vi "4 - extract full movement patterns from XY frame and startend frames.vi"() -> ()   [LabVIEW 2013]
uses:
  <vilib>/Utility/file.llb/Read From Spreadsheet File (DBL).vi
panel:
  in  "XY and frame data 2":path
  in  "Startend":path
  in  "Player position segment data":path
  out "Sub patterns top":string[](array[string])
  out "Sub patterns bottom":string[](array[string])
  out "top":string[](array[string])
  out "bottom":string[](array[string])
  in  "player transition data":dbl[][](array[numeric])=array14018x2[28036 elements] format="%0.3f"
  in  "startend":dbl[][](array[numeric])=[[400.0, 872.0], [1216.0, 1280.0], [1504.0, 1664.0], [2584.0, 2648.0], [2944.0, 3128.0], [3440.0, 3512.0], [3752.0, 4232.0], [4696.0, 4816.0], [5392.0, 5624.0], [6008.0, 6296.0], [6736.0, 7016.0], [7344.0, 7864.0], [8368.0, 8464.0], [8864.0, 8992.0], [9320.0, 9704.0], [11288.0, 11432.0], [11768.0, 11872.0], [12256.0, 12536.0], [12888.0, 13024.0], [13520.0, 13632.0], [13856.0, 14000.0], [14208.0, 14304.0], [14600.0, 14792.0], [15280.0, 15416.0], [15648.0, 15760.0], [16672.0, 16800.0], [17008.0, 17224.0], [17536.0, 17664.0], [17936.0, 18144.0], [18392.0, 18568.0]] format="%0.3f"
  in  "XY and frame data":dbl[][](array[numeric])=array14019x5[70095 elements] format="%0.3f"
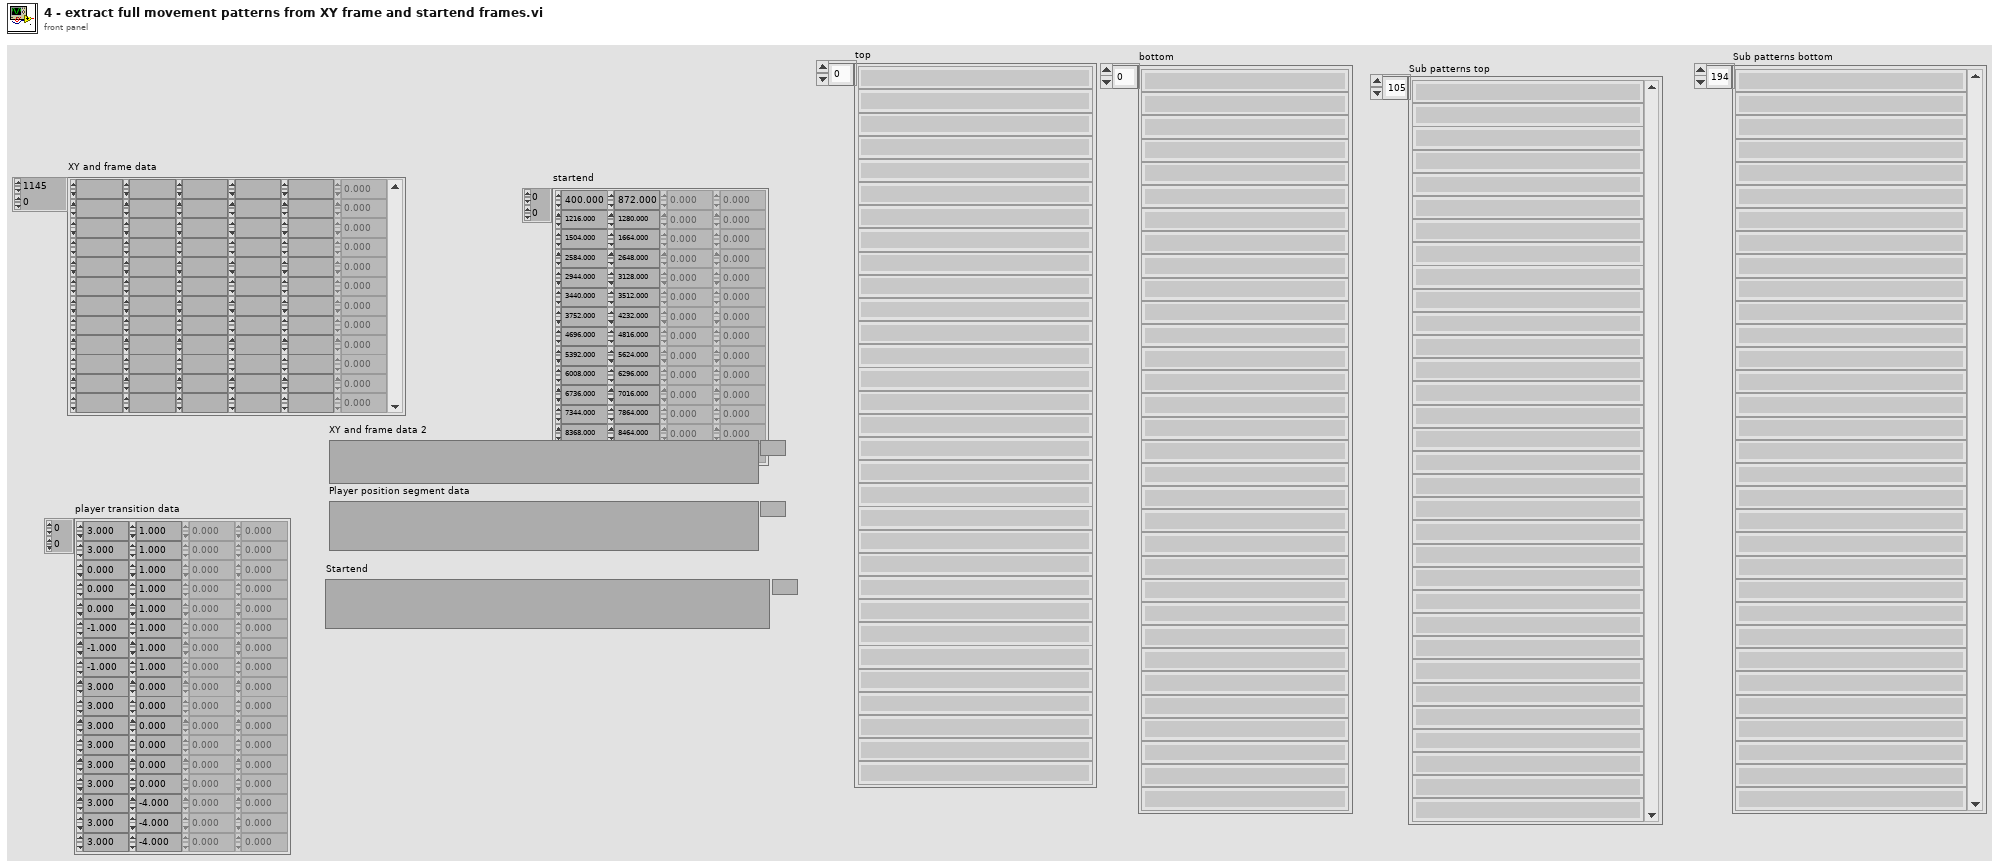
[diagram p1: front panel]
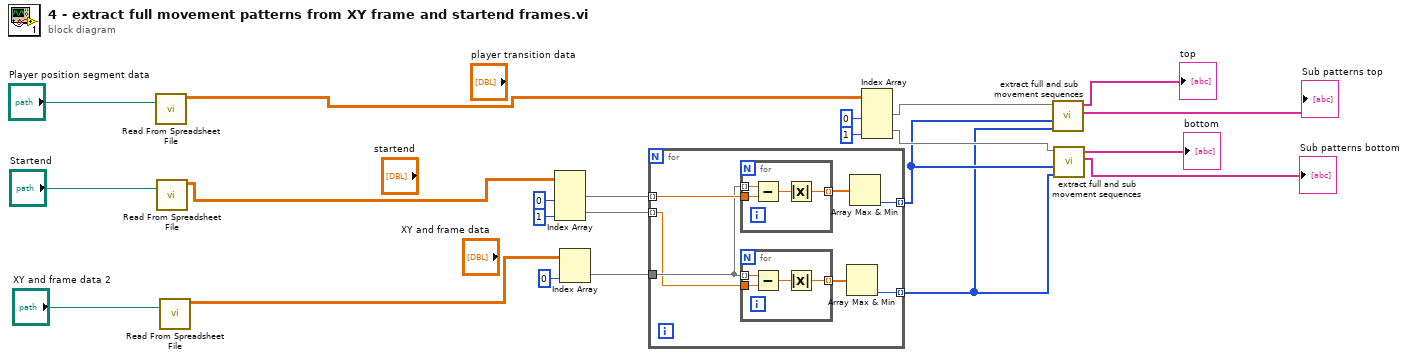
[diagram p0: block diagram]
diagram:
  n1 = call-poly <vilib>:"Read From Spreadsheet File.vi"("file path (dialog if empty)"="Player position segment data") -> ("all rows"=w1:dbl[][])  [unwired: 6 in, 4 out]
  n2 = call-poly <vilib>:"Read From Spreadsheet File.vi"("file path (dialog if empty)"="Startend") -> ("all rows"=w2:dbl[][])  [unwired: 6 in, 4 out]
  n3 = call-poly <vilib>:"Read From Spreadsheet File.vi"("file path (dialog if empty)"="XY and frame data 2") -> ("all rows"=w3:dbl[][])  [unwired: 6 in, 4 out]
  n4 = Index Array(array=w2, index (col) #1=0 ("disabled index (col)"), index (col) #2=1 ("index (col)")) -> (element #1=w20:dbl[], element #2=w19:dbl[])  [unwired: 2 in]
  n5 = Index Array(array=w3, index (col)=0 ("disabled index (col)")) -> (element=w17:dbl[])  [unwired: 1 in]
  n6 = for {
    tunnel: w20 -> [w29] mode=indexing
    tunnel: w19 -> [w24] mode=indexing
    tunnel: w17 -> [w25]
    tunnel: [w27] -> w12 mode=indexing
    tunnel: [w26] -> w11 mode=indexing
    n7 = for {
      tunnel: w29 -> [w36]
      tunnel: w25 -> [w37] mode=indexing
      tunnel: [w34] -> w28 mode=indexing
      n8 = Subtract(x=w37, y=w36) -> (x-y=w35:dbl)
      n9 = Absolute Value(x=w35) -> (abs(x)=w34:dbl)
    }
    n10 = for {
      tunnel: w24 -> [w32]
      tunnel: w25 -> [w33] mode=indexing
      tunnel: [w30] -> w23 mode=indexing
      n11 = Subtract(x=w33, y=w32) -> (x-y=w31:dbl)
      n12 = Absolute Value(x=w31) -> (abs(x)=w30:dbl)
    }
    n13 = Array Max & Min(array=w23) -> (min index (indices)=w26:i32)  [unwired: 3 out]
    n14 = Array Max & Min(array=w28) -> (min index (indices)=w27:i32)  [unwired: 3 out]
  }
  n15 = Index Array(array=w1, index (col) #1=0 ("disabled index (col)"), index (col) #2=1 ("index (col)")) -> (element #1=w14:dbl[], element #2=w13:dbl[])  [unwired: 2 in]
  n16 = call "extract full and sub movement sequences.vi"("end points in"=w11, "Start points in"=w12, "player movement data"=w14) -> ("Sub patterns"=→"Sub patterns top":string[], "Full movement patterns"=→"top":string[])  [unwired: 7 in]
  n17 = call "extract full and sub movement sequences.vi"("end points in"=w11, "Start points in"=w12, "player movement data"=w13) -> ("Sub patterns"=→"Sub patterns bottom":string[], "Full movement patterns"=→"bottom":string[])  [unwired: 7 in]
